vi "ballardTest1553.vi"() -> ()   [LabVIEW 2020]
uses:
  Source/Libraries/Ballard_1553_Parameter_ni/_tyedefs/messageAddress_type.ctl
  Source/Libraries/Ballard_1553_Parameter_ni/_tyedefs/message_type.ctl
  Source/Libraries/Ballard_1553_Parameter_ni/_tyedefs/parameter_type.ctl
  Source/Libraries/Ballard_1553_Parameter_ni/Ballard_1553_Parameter_ni.lvlib
panel:
  in  "parameter configuration":T1={"defaultValue"=0.0, "encoding"=0, "name"="param1", "numberOfBits"=16, "offset"=0.0, "scale"=1.0, "signed"=TRUE, "startBit"=0, "unit"="pascal"} {"encoding" items=["BNR", "BCD", "Discrete"]}
  in  "message configuration":T2={"name"="BC to RT1 (SA2)", "numberOfWords"=1, "modeCode"=0, "messageType"=0, "createTimestampChannel"=TRUE, "modeCodeSpecified"=FALSE} {"messageType" items=["BCtoRT", "RTtoBC", "RTtoRT", "MC"]}
  in  "messageAddresses":T3[](array[typedef])=[{"direction"=1, "subAddress"=2, "terminalAddress"=1}] {"direction" items=["Rx", "Tx"]}
  in  "terminal name":string="BC"
  in  "terminalAddress":i32
  in  "hardwareChannel":i32
  in  "XML path":path=path "C:/Users/Administrator/Desktop/GIT/Ballard-Arinc-429-XML-Generator/Database Examples/ParametersBallard_1553.xml"
  out "error out":errorcluster
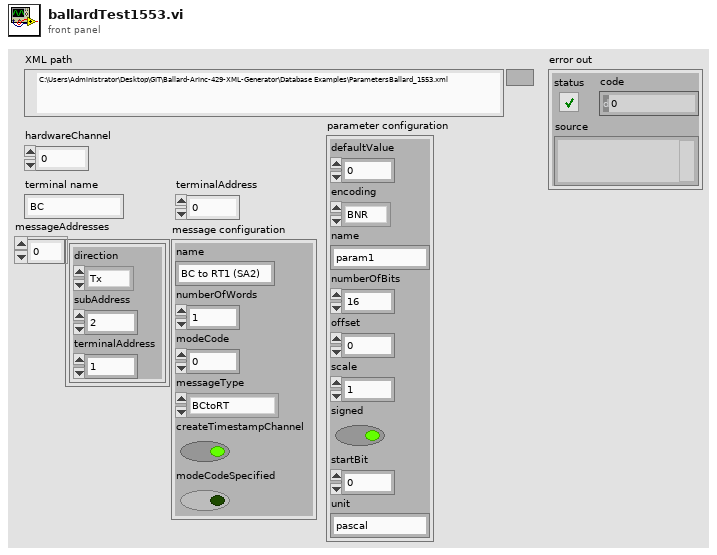
[diagram p1: front panel]
types:
  T1 = typedef "Ballard_1553_Parameter_ni.lvlib/parameter_type.ctl" = cluster{"defaultValue":dbl, "encoding":i32, "name":string, "numberOfBits":i32, "offset":dbl, "scale":dbl, "signed":bool, "startBit":i32, "unit":string}
  T2 = typedef "Ballard_1553_Parameter_ni.lvlib/message_type.ctl" = cluster{"name":string, "numberOfWords":i32, "modeCode":i32, "messageType":i32, "createTimestampChannel":bool, "modeCodeSpecified":bool}
  T3 = typedef "Ballard_1553_Parameter_ni.lvlib/messageAddress_type.ctl" = cluster{"direction":i32, "subAddress":i32, "terminalAddress":i32}
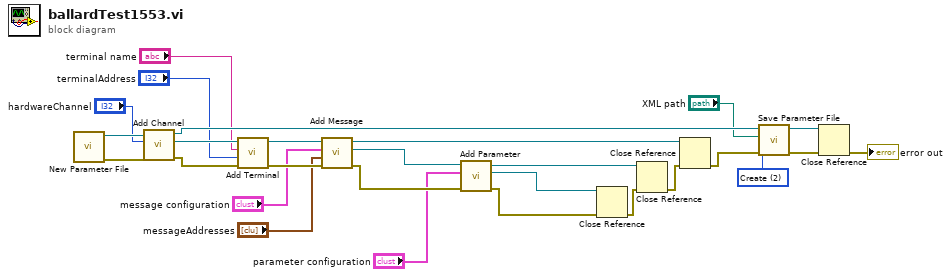
[diagram p0: block diagram]
diagram:
  w7 = 2 items=["CreateNew"=1, "Create"=2, "Open"=3, "OpenOrCreate"=4, "Truncate"=5, "Append"=6] ("mode (Create)")
  n1 = call "New Parameter File.vi"() -> ("error out"=w26:errorcluster, "new parameter file"=w27:refnum<k24>)  [unwired: 10 in]
  n2 = call "Add Channel.vi"("error in"=w26, "hardwareChannel"="hardwareChannel", "parameter file in"=w27) -> ("error out"=w25:errorcluster, "new channel"=w21:refnum<k24>, "parameter file out"=w22:refnum<k24>)  [unwired: 6 in]
  n3 = call "Add Terminal.vi"("error in"=w25, "terminalAddress"="terminalAddress", "name"="terminal name", "channel in"=w21) -> ("error out"=w23:errorcluster, "channel out"=w24:refnum<k24>)  [unwired: 5 in, 1 out]
  n4 = call "Add Message.vi"("error in"=w23, "messageAddresses"="messageAddresses", "message configuration"="message configuration", "channel in"=w24) -> ("error out"=w19:errorcluster, "new message"=w20:refnum<k24>, "channel out"=w14:refnum<k24>)  [unwired: 5 in]
  n5 = call "Add Parameter.vi"("error in"=w19, "parameter configuration"="parameter configuration", "message in"=w20) -> ("error out"=w9:errorcluster, "new parameter"=w11:refnum<k24>, "message out"=w12:refnum<k24>)  [unwired: 6 in]
  n6 = Close Reference(reference=w11, error in (no error)=w9) -> (error out=w10:errorcluster)
  n7 = Close Reference(reference=w12, error in (no error)=w10) -> (error out=w15:errorcluster)
  n8 = Close Reference(reference=w14, error in (no error)=w15) -> (error out=w13:errorcluster)
  n9 = call "Save Parameter File.vi"("error in"=w13, "mode (Create)"=w7, "XML path"="XML path", "parameter file in"=w22) -> ("error out"=w18:errorcluster, "parameter file out"=w16:refnum<k24>)  [unwired: 5 in, 1 out]
  n10 = Close Reference(reference=w16, error in (no error)=w18) -> (error out=→"error out":errorcluster)
